vi "ReadDisplayConfiguration.vi"(8 "Error In":errorcluster, 11 "ABLE Config File Ref In":T2) -> (0 "Error Out":errorcluster, 2 "Display Configuration":T1, 3 "ABLE Config File Ref Out":T2)   [LabVIEW 2012]
uses:
  <vilib>/Utility/config.llb/Config Data RefNum.ctl
  DisplayConfiguration.ctl
  <vilib>/Utility/config.llb/Read Key (U32).vi
  <vilib>/Utility/config.llb/Read Key (Boolean).vi
  <vilib>/Utility/config.llb/NI_LVConfig.lvlib
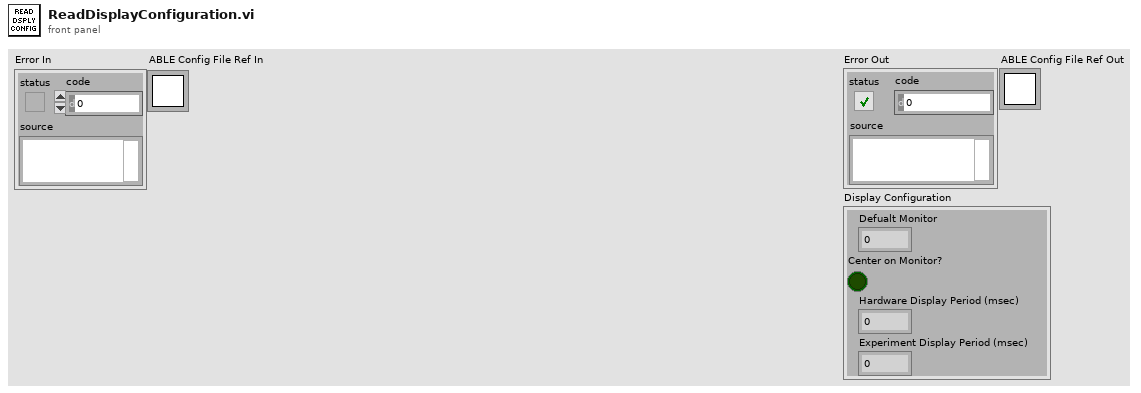
[diagram p1: front panel]
types:
  T1 = typedef "DisplayConfiguration.ctl" = cluster{"Defualt Monitor":u16, "Center on Monitor?":bool, "Hardware Display Period (msec)":u32, "Experiment Display Period (msec)":u32}
  T2 = typedef "NI_LVConfig.lvlib/Config Data RefNum.ctl" = refnum<k1>
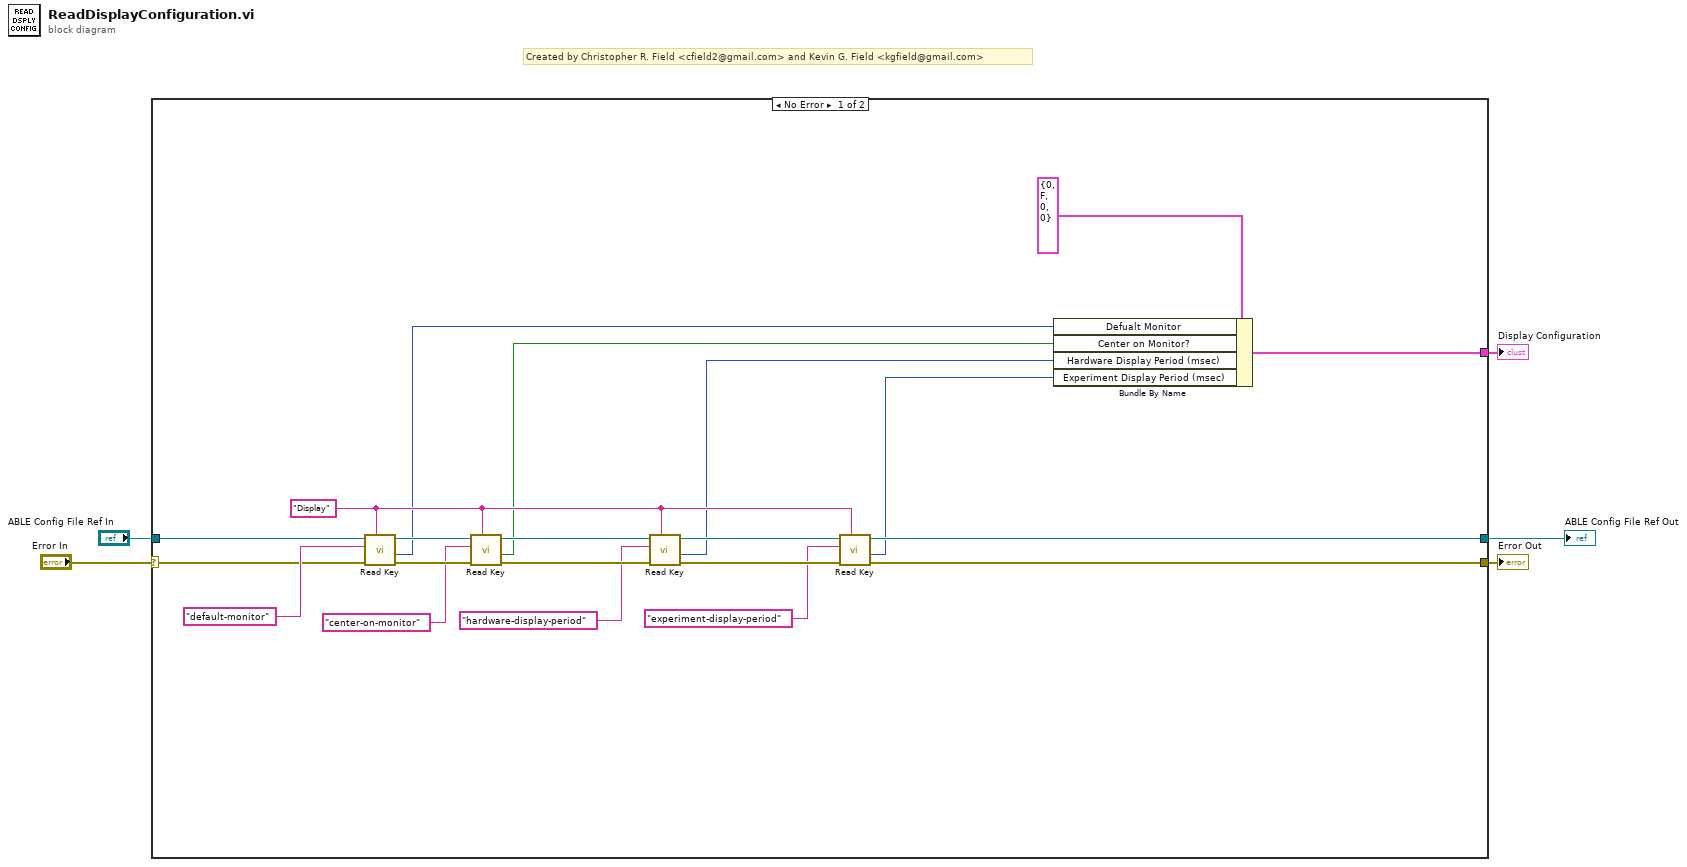
[diagram p0: block diagram]
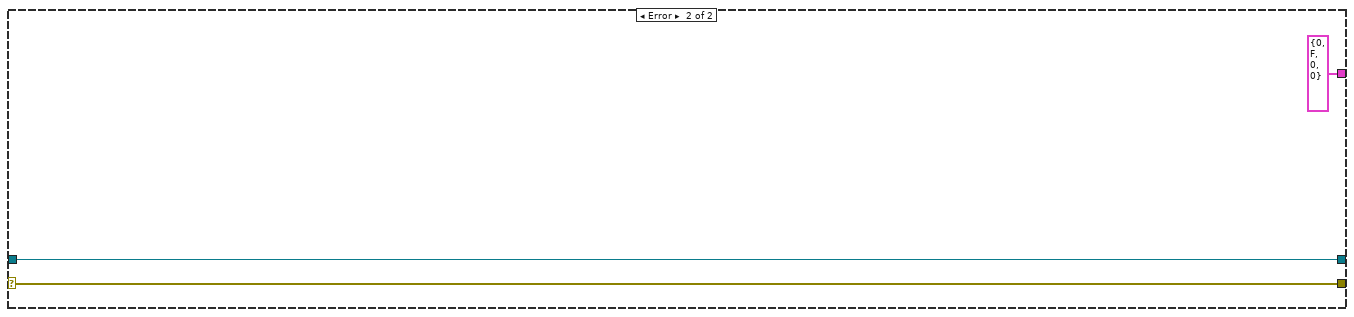
[diagram p2: hidden frame]
diagram:
  # "Created by Christopher R. Field <cfield2@gmail.com> and Kevin G. Field <kgfield@gmail.com>"
  n1 = case shown="No Error" "Error In" {
    selector: "Error In" -> [w22 w28]
    tunnel: "ABLE Config File Ref In" -> [w21 w29]
    tunnel: [w13 w28] -> w3
    tunnel: [w12 w29] -> w2
    tunnel: [w6 T1 {"Defualt Monitor"=0, "Center on Monitor?"=FALSE, "Hardware Display Period (msec)"=0, "Experiment Display Period (msec)"=0} ("Display Configuration")] -> w1
    frame No Error {
      w15 = "Display" ("section")
      n2 = call-poly <vilib>:"Read Key.vi"("section"=w15, "error in (no error)"=w22, "key"="default-monitor", "refnum"=w21) -> ("error out"=w25:errorcluster, "value"=w10:u32, "refnum out"=w26:T2)  [unwired: 4 in, 1 out]
      n3 = call-poly <vilib>:"Read Key.vi"("section"=w15, "error in (no error)"=w25, "key"="center-on-monitor", "refnum"=w26) -> ("error out"=w19:errorcluster, "value"=w9:bool, "refnum out"=w20:T2)  [unwired: 4 in, 1 out]
      n4 = call-poly <vilib>:"Read Key.vi"("section"=w15, "error in (no error)"=w19, "key"="hardware-display-period", "refnum"=w20) -> ("error out"=w16:errorcluster, "value"=w8:u32, "refnum out"=w17:T2)  [unwired: 4 in, 1 out]
      n5 = call-poly <vilib>:"Read Key.vi"("section"=w15, "error in (no error)"=w16, "key"="experiment-display-period", "refnum"=w17) -> ("error out"=w13:errorcluster, "value"=w7:u32, "refnum out"=w12:T2)  [unwired: 4 in, 1 out]
      n6 = Bundle By Name(cluster=T1 {"Defualt Monitor"=0, "Center on Monitor?"=FALSE, "Hardware Display Period (msec)"=0, "Experiment Display Period (msec)"=0} ("Display Configuration"), "Defualt Monitor"=w10, "Center on Monitor?"=w9, "Hardware Display Period (msec)"=w8, "Experiment Display Period (msec)"=w7) -> (w6:T1)
    }
    frame Error {
    }
  }
  "Error Out" <- w3
  "ABLE Config File Ref Out" <- w2
  "Display Configuration" <- w1
